vi "WSVCAP SHL Host LL SPI Convert Channel Bytes to Bit Array.vi"(0 "SPI Data [DUT Ordered]":u8[][](array[numeric]) format="%02x", 7 "Cycle CMD Lengths Out (bits)":u8[](array[numeric]), 9 "Cycle CMD Delay Out (ticks)":u32[](array[numeric])) -> (4 "Write Data":u64[](array[numeric]) format="%016x")   [LabVIEW 2012]
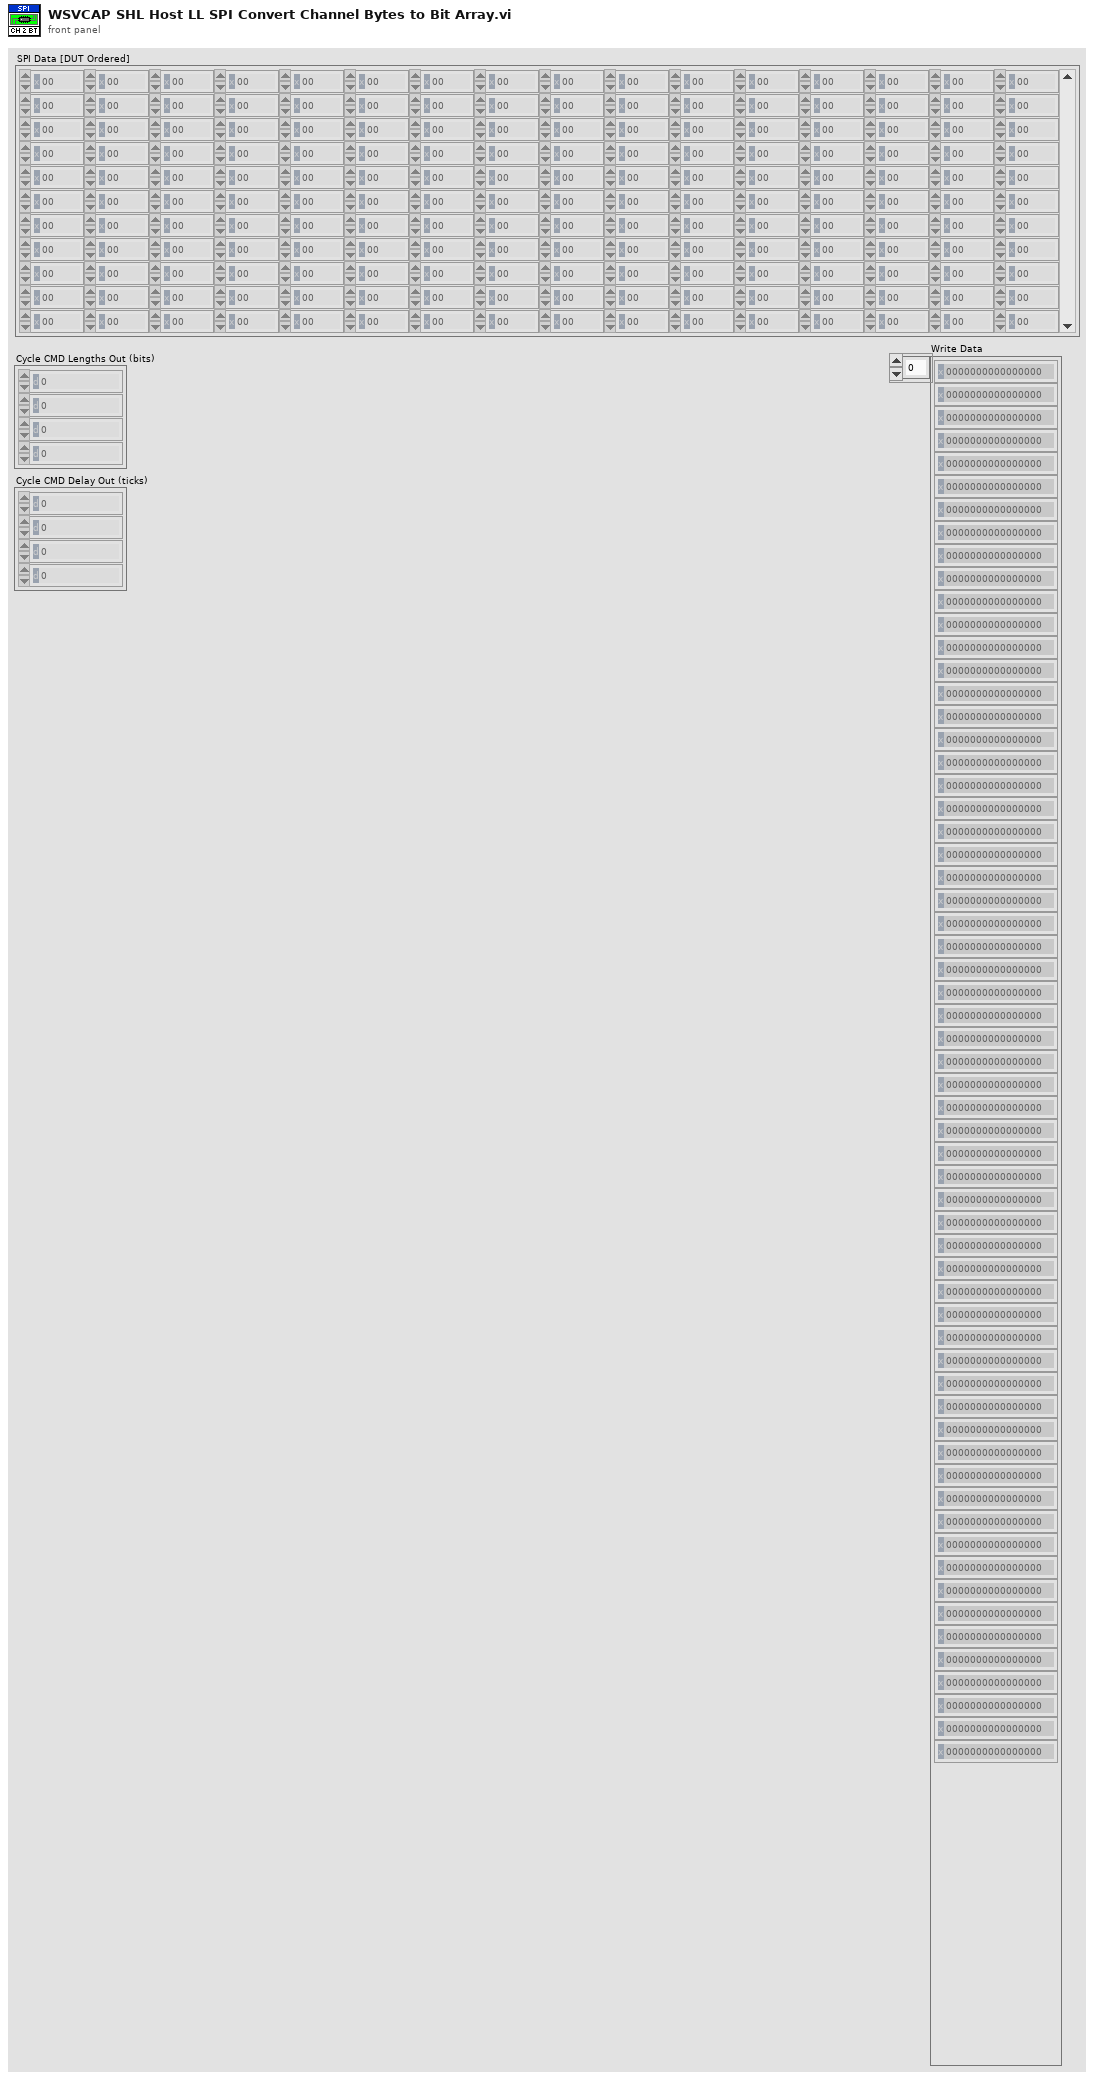
[diagram p1: front panel]
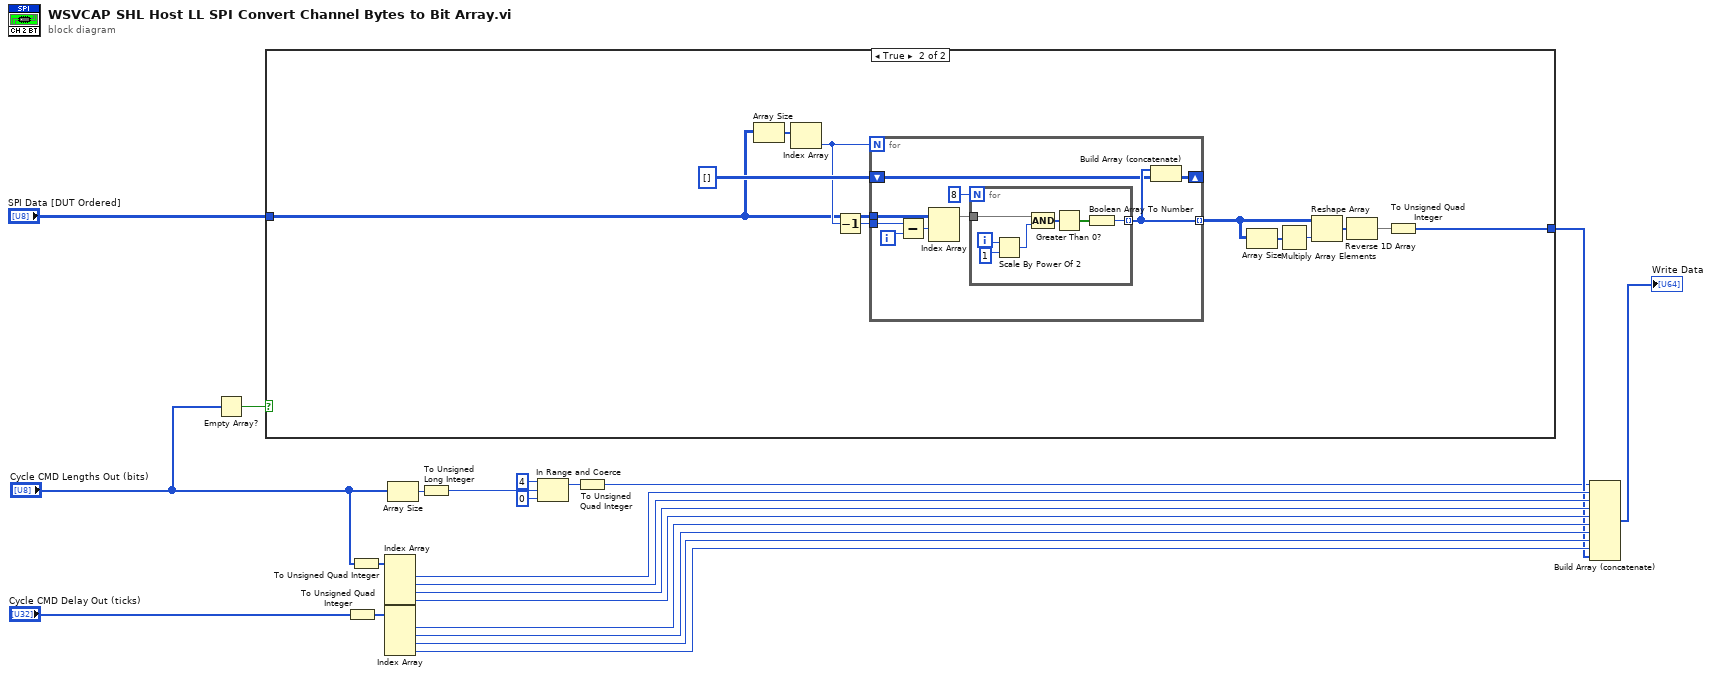
[diagram p0: block diagram]
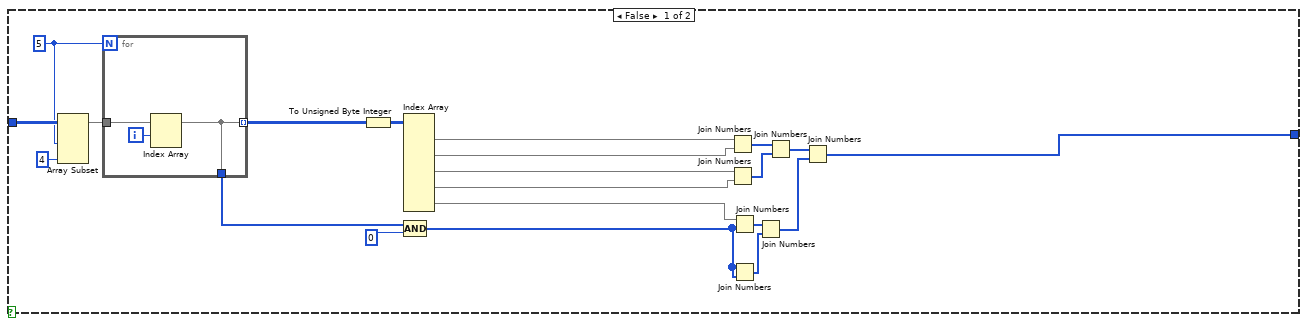
[diagram p2: hidden frame]
diagram:
  n1 = Empty Array?(array="Cycle CMD Lengths Out (bits)") -> (empty?=w3:bool)
  n2 = case shown="True" w3 {
    tunnel: "SPI Data [DUT Ordered]" -> [w29 w47]
    tunnel: [w36 w48] -> w5
    frame False {
      w27 = 5
      n3 = Array Subset(array=w29, length (row)=w27, length (col)=4 ("length")) -> (w28:u8[][])  [unwired: 2 in]
      n4 = for {
        N: w27 -> [_]
        tunnel: w28 -> [w46]
        tunnel: [w44] -> w30 mode=indexing
        tunnel: [w44] -> w25
        i -> [w45]
        n5 = Index Array(array=w46, index (row)=w45) -> (element=w44:u8[])  [unwired: 1 in]
      }
      n6 = To Unsigned Byte Integer(number=w30) -> (unsigned 8bit integer=w35:u8[][])
      n7 = Index Array(array=w35) -> (element #1=w43:u8[], element #2=w42:u8[], element #3=w41:u8[], element #4=w40:u8[], element #5=w34:u8[])  [unwired: 10 in]
      n8 = Compound Arithmetic op=AND(w25, u8 0 ("Read Data")) -> (w24:u8[])
      n9 = Join Numbers(hi=w43, lo=w42) -> ((hi.lo)=w39:u16[])
      n10 = Join Numbers(hi=w41, lo=w40) -> ((hi.lo)=w38:u16[])
      n11 = Join Numbers(hi=w34, lo=w24) -> ((hi.lo)=w33:u16[])
      n12 = Join Numbers(hi=w24, lo=w24) -> ((hi.lo)=w32:u16[])
      n13 = Join Numbers(hi=w33, lo=w32) -> ((hi.lo)=w31:u32[])
      n14 = Join Numbers(hi=w39, lo=w38) -> ((hi.lo)=w37:u32[])
      n15 = Join Numbers(hi=w37, lo=w31) -> ((hi.lo)=w36:u64[])
    }
    frame True {
      n16 = Array Size(array=w47) -> (size(s)=w53:i32[])
      n17 = Index Array(array=w53) -> (element=w51:i32)  [unwired: 1 in]
      n18 = Decrement(x=w51) -> (x-1=w50:i32)
      n19 = for {
        N: w51 -> [_]
        tunnel: w47 -> [w62]
        tunnel: [w65] -> w57 mode=indexing
        shift-right: [w64] -> _
        shift-left: u32[][] [] -> [w63]
        tunnel: w50 -> [w58]
        i -> [w60]
        n20 = Subtract(x=w58, y=w60) -> (x-y=w59:i32)
        n21 = Index Array(array=w62, index (row)=w59) -> (element=w61:u8[])  [unwired: 1 in]
        n22 = for {
          N: 8 -> [_]
          tunnel: w61 -> [w69]
          tunnel: [w68] -> w65 mode=indexing
          i -> [w71]
          n23 = Scale By Power Of 2(n=w71, x=u8 1) -> (x*2^n=w72:u8)
          n24 = Compound Arithmetic op=AND(w69, w72) -> (w73:u8[])
          n25 = Greater Than 0?(x=w73) -> (x > 0?=w67:bool[])
          n26 = Boolean Array To Number(Boolean array=w67) -> (number=w68:u32)
        }
        n27 = Build Array (concatenate)(w65, w63) -> (w64:u32[][])
      }
      n28 = Array Size(array=w57) -> (size(s)=w56:i32[])
      n29 = Multiply Array Elements(1:w56) -> (0:w55:i32)
      n30 = Reshape Array(w57, w55) -> (w52:u32[])
      n31 = Reverse 1D Array(array=w52) -> (reversed array=w49:u32[])
      n32 = To Unsigned Quad Integer(1:w49) -> (0:w48:u64[])
    }
  }
  n33 = To Unsigned Quad Integer(1:"Cycle CMD Delay Out (ticks)") -> (0:w2:u64[])
  n34 = To Unsigned Quad Integer(1:"Cycle CMD Lengths Out (bits)") -> (0:w14:u64[])
  n35 = Index Array(array=w14) -> (element #1=w16:u64, element #2=w15:u64, element #3=w13:u64, element #4=w12:u64)  [unwired: 4 in]
  n36 = Index Array(array=w2) -> (element #1=w11:u64, element #2=w10:u64, element #3=w9:u64, element #4=w8:u64)  [unwired: 4 in]
  n37 = Array Size(array="Cycle CMD Lengths Out (bits)") -> (size(s)=w21:i32)
  n38 = To Unsigned Long Integer(number=w21) -> (unsigned 32bit integer=w6:u32)
  n39 = In Range and Coerce(upper limit=u32 4, x=w6, lower limit=u32 0) -> (coerced(x)=w18:u32)  [unwired: 1 out]
  n40 = To Unsigned Quad Integer(1:w18) -> (0:w1:u64)
  n41 = Build Array (concatenate)(w1, w16, w15, w13, w12, w11, w10, w9, w8, w5) -> (→"Write Data":u64[])
